vi "Test Copy from Pixmap Greyscale.vi"(8 "error in (no error)":errorcluster, 11 "Test Case In":refnum<class "Image.lvclass">) -> (0 "error out":errorcluster, 3 "Test Case Out":refnum<class "Image.lvclass">)   [LabVIEW 2020, in "g_ar_toolkit.test.lvlib" / "Image.lvclass"]
uses:
  Image.lvclass
  C:/Program Files (x86)/National Instruments/LabVIEW 2020/vi.lib/Astemes/LUnit/Test Case.lvclass
  <vilib>/picture/picture.llb/imagedata.ctl
  <vilib>/Astemes/LUnit/Test Case.lvclass/Test Case.ctl
  2c93f62b-78d7-4b59-b27c-14bd701a5d71.vi
  8166983f-db3b-480f-a786-a958408166cb.vi
  03fde0f0-e029-4dad-9f9a-a95d25ce423a.vi
  3bb2986f-6074-4300-8ef6-a7ee1c3ba308.vi
  02fb1d00-84d2-4392-bb0c-78c1f80e642d.vi
  g_ar_toolkit.image/CreateEmptyImageGreyscale.vi
  g_ar_toolkit.image/CopyPixmapToImageOuptutMaskGreyscale.vi
  g_ar_toolkit.image/CopyPixmapToImageIgnoreMaskGreyscale.vi
  7f5bb767-9dbf-47d9-8f44-5f4901e96d00.vi
  e6d5ae8e-bd70-4c65-a769-b7cfb03e80c7.vi
  d454bffa-6717-48ab-b8d5-b1f03345aa55.vi
  g_ar_toolkit.image/CreateEmptyImageGreyscale.vi/6598b9e0-8a08-46f5-91fd-ca1b87217137.vi
  g_ar_toolkit.image/CopyPixmapToImageOuptutMaskGreyscale.vi/80b1166a-8c06-443b-b271-eb6a715622f7.vi
  g_ar_toolkit.image/CopyPixmapToImageIgnoreMaskGreyscale.vi/80b1166a-8c06-443b-b271-eb6a715622f7.vi
  <vilib>/Astemes/LUnit/Append Pass Result.vi
  <vilib>/Astemes/LUnit/Append Fail Result.vi
  <vilib>/Astemes/LUnit/Describe Comparison.vi
  <vilib>/Astemes/LUnit/Compare Variants.vi
  g_ar_toolkit.image/FixPixmapColourArraySize.vi
  <vilib>/Astemes/LUnit/Variant to string.vi
  g_ar_toolkit.image/Default8bitColourMap.vi
  <vilib>/Utility/colorconv.llb/Color to RGB.vi
  <vilib>/Utility/error.llb/Error Cluster From Error Code.vi
  <vilib>/Utility/Data Type/Get Type Information.vi
  <vilib>/Utility/LVClass/Get LV Class Name.vi
  g_ar_toolkit.image/g_ar_toolkit.image.lvlib
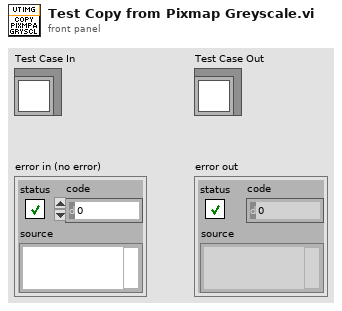
[diagram p1: front panel]
types:
  T1 = enum16{"8 Bit No Mask", "24 Bit No Mask", "32 Bit No Mask", "8 Bit Mask", "24 Bit Mask", "32 Bit Mask", "8 Pixels Wide Masked", "16 Pixels Wide Masked"}
  T2 = typedef "imagedata.ctl" = cluster{"image type":i32, "image depth":i32, "image":u8[], "mask":u8[], "colors":u32[], "Rectangle":cluster{"left":i16, "top":i16, "right":i16, "bottom":i16}}
  T3 = cluster{"8 No Mask":T2, "8 Mask":T2, "24 No Mask":T2, "24 Mask":T2, "32 No Mask":T2, "32 Mask":T2, "24 Mask - 8 wide":T2, "24 Mask - 16 wide":T2}
  T4 = cluster{"left":i16, "top":i16, "right":i16, "bottom":i16}
  T5 = enum16{"8 Bit No Mask", "24 Bit No Mask", "32 Bit No Mask", "8 Bit Mask", "24 Bit Mask", "32 Bit Mask", "8 Pixels Wide Masked", "16 Pixels Wide Masked"}[]
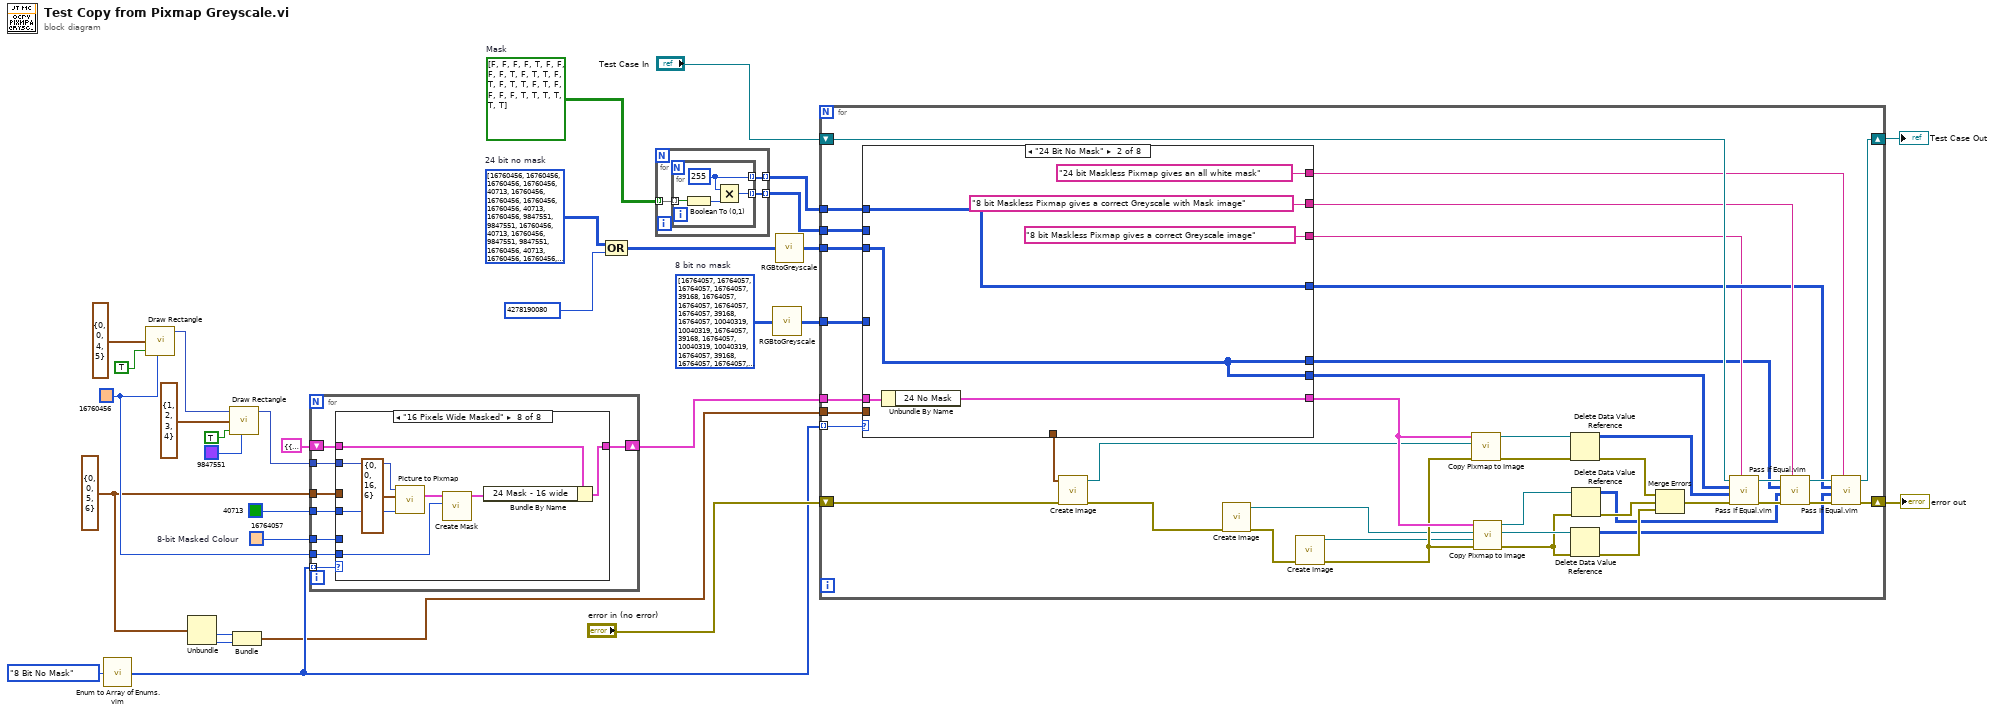
[diagram p0: block diagram]
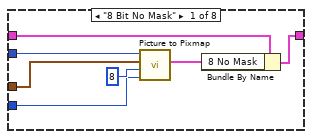
[diagram p2: hidden frame]
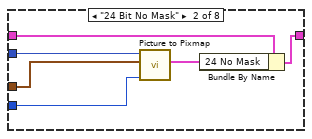
[diagram p3: hidden frame]
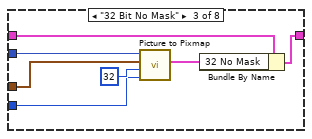
[diagram p4: hidden frame]
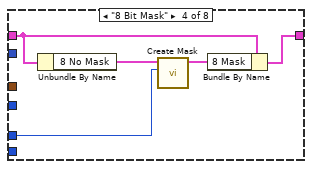
[diagram p5: hidden frame]
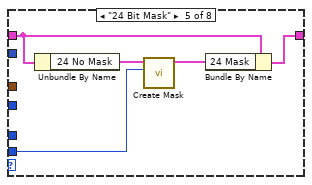
[diagram p6: hidden frame]
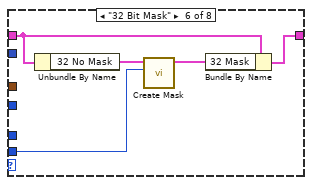
[diagram p7: hidden frame]
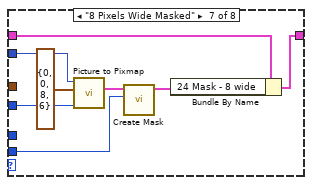
[diagram p8: hidden frame]
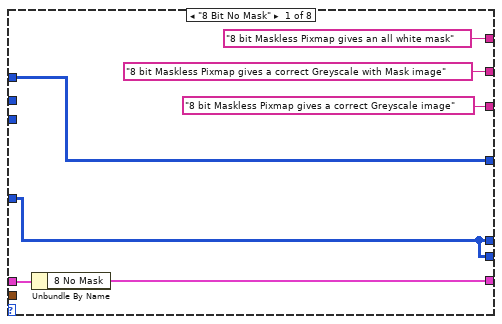
[diagram p9: hidden frame]
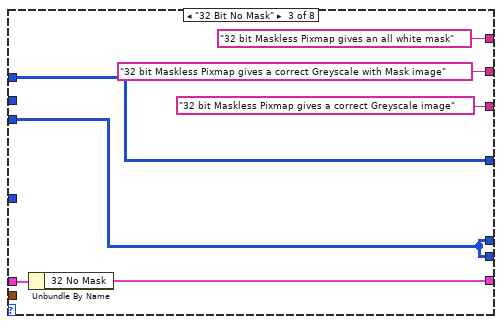
[diagram p10: hidden frame]
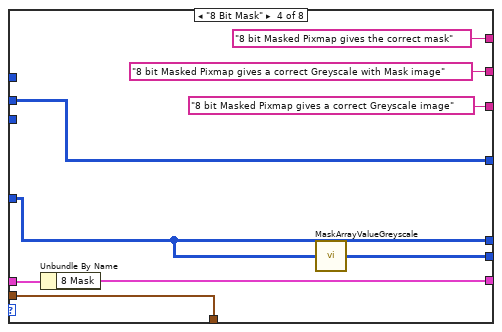
[diagram p11: hidden frame]
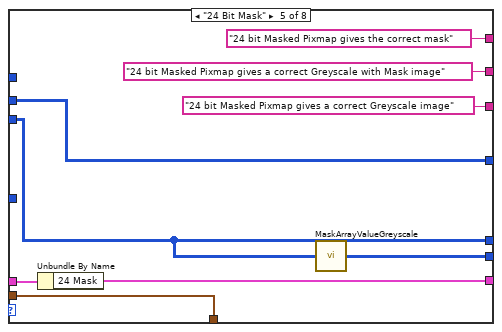
[diagram p12: hidden frame]
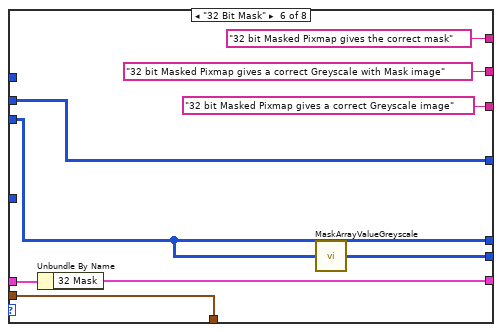
[diagram p13: hidden frame]
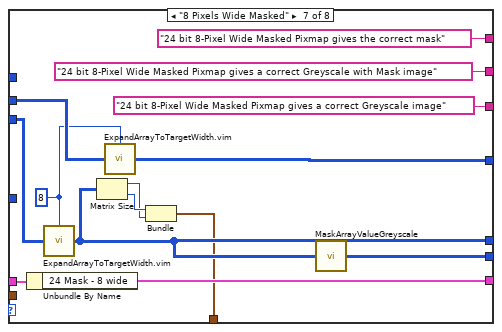
[diagram p14: hidden frame]
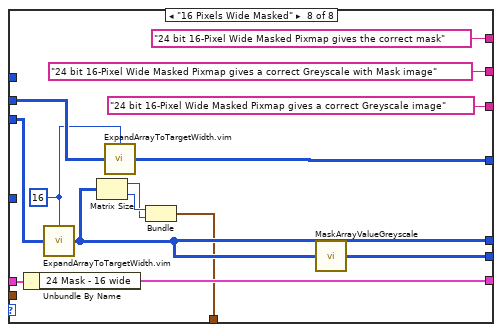
[diagram p15: hidden frame]
diagram:
  w5 = u32 16764057  # 8-bit Masked Colour
  w18 = bool[][] [[FALSE, FALSE, FALSE, FALSE, TRUE], [FALSE, FALSE, FALSE, FALSE, TRUE], [FALSE, TRUE, TRUE, FALSE, TRUE], [FALSE, TRUE, TRUE, FALSE, TRUE], [FALSE, FALSE, FALSE, FALSE, TRUE], [TRUE, TRUE, TRUE, TRUE, TRUE]]  # Mask
  w2 = u32[][] [[16764057, 16764057, 16764057, 16764057, 39168], [16764057, 16764057, 16764057, 16764057, 39168], [16764057, 10040319, 10040319, 16764057, 39168], [16764057, 10040319, 10040319, 16764057, 39168], [16764057, 16764057, 16764057, 16764057, 39168], [39168, 39168, 39168, 39168, 39168]]  # 8 bit no mask
  w21 = u32[][] [[16760456, 16760456, 16760456, 16760456, 40713], [16760456, 16760456, 16760456, 16760456, 40713], [16760456, 9847551, 9847551, 16760456, 40713], [16760456, 9847551, 9847551, 16760456, 40713], [16760456, 16760456, 16760456, 16760456, 40713], [40713, 40713, 40713, 40713, 40713]]  # 24 bit no mask
  w9 = T4 {"left"=0, "top"=0, "right"=5, "bottom"=6} ("rect")
  w12 = u32 16760456 ("color(black)")
  n1 = call "Enum to Array of Enums.vim"("enum"=T1."8 Bit No Mask") -> ("array of enums"=w16:T5)
  n2 = call <vilib>:"Draw Rectangle.vi"("rect"=T4 {"left"=0, "top"=0, "right"=4, "bottom"=5}, "fill?(F)"=TRUE, "color(black)"=w12) -> ("new picture"=w31:picture)  [unwired: 6 in]
  n3 = Unbundle(w9) -> ("right"=w8:i16, "bottom"=w7:i16)  [unwired: 2 out]
  n4 = call <vilib>:"Draw Rectangle.vi"("picture"=w31, "rect"=T4 {"left"=1, "top"=2, "right"=3, "bottom"=4}, "fill?(F)"=TRUE, "color(black)"=u32 9847551) -> ("new picture"=w13:picture)  [unwired: 5 in]
  n5 = Bundle("right"=w8, "bottom"=w7) -> (w6:cluster{"right":i16, "bottom":i16})  [unwired: 1 in]
  n6 = for {
    tunnel: w16 -> [w37] mode=indexing
    shift-right: [w38] -> w14
    shift-left: T3 {"8 No Mask"={"image type"=0, "image depth"=0, "image"=[], "mask"=[], "colors"=[], "Rectangle"={"left"=0, "top"=0, "right"=0, "bottom"=0}}, "8 Mask"={"image type"=0, "image depth"=0, "image"=[], "mask"=[], "colors"=[], "Rectangle"={"left"=0, "top"=0, "right"=0, "bottom"=0}}, "24 No Mask"={"image type"=0, "image depth"=0, "image"=[], "mask"=[], "colors"=[], "Rectangle"={"left"=0, "top"=0, "right"=0, "bottom"=0}}, "24 Mask"={"image type"=0, "image depth"=0, "image"=[], "mask"=[], "colors"=[], "Rectangle"={"left"=0, "top"=0, "right"=0, "bottom"=0}}, "32 No Mask"={"image type"=0, "image depth"=0, "image"=[], "mask"=[], "colors"=[], "Rectangle"={"left"=0, "top"=0, "right"=0, "bottom"=0}}, "32 Mask"={"image type"=0, "image depth"=0, "image"=[], "mask"=[], "colors"=[], "Rectangle"={"left"=0, "top"=0, "right"=0, "bottom"=0}}, "24 Mask - 8 wide"={"image type"=0, "image depth"=0, "image"=[], "mask"=[], "colors"=[], "Rectangle"={"left"=0, "top"=0, "right"=0, "bottom"=0}}, "24 Mask - 16 wide"={"image type"=0, "image depth"=0, "image"=[], "mask"=[], "colors"=[], "Rectangle"={"left"=0, "top"=0, "right"=0, "bottom"=0}}} ("output cluster") -> [w39]
    tunnel: w13 -> [w35]
    tunnel: w9 -> [w36]
    tunnel: u32 40713 ("Background Color") -> [w34]
    tunnel: w12 -> [w33]
    tunnel: w5 -> [w32]
    n7 = case shown="\"16 Pixels Wide Masked\"" w37 {
      tunnel: w39 -> [w46 w52 w59 w63 w68 w73 w82 w90]
      tunnel: [w45 w51 w58 w64 w69 w74 w81 w89] -> w38
      tunnel: w36 -> [w43 w50 w56 _ _ _ _ _]
      tunnel: w35 -> [w42 w49 w55 _ _ _ w78 w86]
      tunnel: w34 -> [w40 w47 w53 _ _ _ w77 w85]
      tunnel: w33 -> [_ _ _ _ w65 w70 w75 w83]
      tunnel: w32 -> [_ _ _ w60 _ _ _ _]
      frame "8 Bit No Mask" {
        n8 = call <vilib>:"Picture to Pixmap.vi"("Background Color"=w40, "depth"=8, "rect"=w43, "picture"=w42) -> ("image data"=w41:T2)  [unwired: 6 in, 1 out]
        n9 = Bundle By Name(cluster=w46, "8 No Mask"=w41) -> (w45:T3)
      }
      frame "24 Bit No Mask" {
        n10 = call <vilib>:"Picture to Pixmap.vi"("Background Color"=w47, "rect"=w50, "picture"=w49) -> ("image data"=w48:T2)  [unwired: 7 in, 1 out]
        n11 = Bundle By Name(cluster=w52, "24 No Mask"=w48) -> (w51:T3)
      }
      frame "32 Bit No Mask" {
        n12 = call <vilib>:"Picture to Pixmap.vi"("Background Color"=w53, "depth"=32, "rect"=w56, "picture"=w55) -> ("image data"=w54:T2)  [unwired: 6 in, 1 out]
        n13 = Bundle By Name(cluster=w59, "32 No Mask"=w54) -> (w58:T3)
      }
      frame "8 Bit Mask" {
        n14 = Unbundle By Name(w63) -> ("8 No Mask"=w62:T2)
        n15 = call <vilib>:"Create Mask.vi"("Mask Color (Black)"=w60, "image data"=w62) -> ("image data"=w61:T2)  [unwired: 9 in]
        n16 = Bundle By Name(cluster=w63, "8 Mask"=w61) -> (w64:T3)
      }
      frame "24 Bit Mask" {
        n17 = Unbundle By Name(w68) -> ("24 No Mask"=w67:T2)
        n18 = call <vilib>:"Create Mask.vi"("Mask Color (Black)"=w65, "image data"=w67) -> ("image data"=w66:T2)  [unwired: 9 in]
        n19 = Bundle By Name(cluster=w68, "24 Mask"=w66) -> (w69:T3)
      }
      frame "32 Bit Mask" {
        n20 = Unbundle By Name(w73) -> ("32 No Mask"=w72:T2)
        n21 = call <vilib>:"Create Mask.vi"("Mask Color (Black)"=w70, "image data"=w72) -> ("image data"=w71:T2)  [unwired: 9 in]
        n22 = Bundle By Name(cluster=w73, "32 Mask"=w71) -> (w74:T3)
      }
      frame "8 Pixels Wide Masked" {
        n23 = call <vilib>:"Picture to Pixmap.vi"("Background Color"=w77, "rect"=T4 {"left"=0, "top"=0, "right"=8, "bottom"=6}, "picture"=w78) -> ("image data"=w80:T2)  [unwired: 7 in, 1 out]
        n24 = call <vilib>:"Create Mask.vi"("Mask Color (Black)"=w75, "image data"=w80) -> ("image data"=w79:T2)  [unwired: 9 in]
        n25 = Bundle By Name(cluster=w82, "24 Mask - 8 wide"=w79) -> (w81:T3)
      }
      frame "16 Pixels Wide Masked" {
        n26 = call <vilib>:"Picture to Pixmap.vi"("Background Color"=w85, "rect"=T4 {"left"=0, "top"=0, "right"=16, "bottom"=6}, "picture"=w86) -> ("image data"=w88:T2)  [unwired: 7 in, 1 out]
        n27 = call <vilib>:"Create Mask.vi"("Mask Color (Black)"=w83, "image data"=w88) -> ("image data"=w87:T2)  [unwired: 9 in]
        n28 = Bundle By Name(cluster=w90, "24 Mask - 16 wide"=w87) -> (w89:T3)
      }
    }
  }
  n29 = Compound Arithmetic op=OR(w21, u32 4278190080) -> (w20:u32[][])
  n30 = for "Masks" {
    tunnel: w18 -> [w92] mode=indexing
    tunnel: [w93] -> w19 mode=indexing
    tunnel: [w91] -> w17 mode=indexing
    n31 = for {
      tunnel: [w96] -> w93 mode=indexing
      tunnel: w92 -> [w97] mode=indexing
      tunnel: [w95] -> w91 mode=indexing
      w96 = u8 255 ("unsigned 8bit integer")
      n32 = Boolean To (0,1)(Boolean=w97) -> (0, 1=w94:i16)
      n33 = Multiply(x=w96, y=w94) -> (x*y=w95:u8)
    }
  }
  n34 = call "RGBtoGreyscale.vi"("RBG"=w2) -> ("Greyscale"=w3:u8[][])
  n35 = call "RGBtoGreyscale.vi"("RBG"=w20) -> ("Greyscale"=w1:u8[][])
  n36 = for {
    tunnel: w14 -> [w138]
    tunnel: w16 -> [w132] mode=indexing
    shift-right: [w123] -> w22
    shift-left: "error in (no error)" -> [w115]
    shift-right: [w122] -> w25
    shift-left: "Test Case In" -> [w131]
    tunnel: w1 -> [w116]
    tunnel: w3 -> [w119]
    tunnel: w19 -> [w112]
    tunnel: w17 -> [w111]
    tunnel: w6 -> [w106]
    n37 = case shown="\"24 Bit No Mask\"" w132 {
      tunnel: w138 -> [w145 w152 w159 w168 w177 w186 w200 w214]
      tunnel: [w144 w151 w158 w167 w176 w185 w199 w213] -> w137
      tunnel: ["8 bit Maskless Pixmap gives an all white mask" ("Description") "24 bit Maskless Pixmap gives an all white mask" ("Description") "32 bit Maskless Pixmap gives an all white mask" ("Description") "8 bit Masked Pixmap gives the correct mask" ("Description") "24 bit Masked Pixmap gives the correct mask" ("Description") "32 bit Masked Pixmap gives the correct mask" ("Description") "24 bit 8-Pixel Wide Masked Pixmap gives the correct mask" ("Description") "24 bit 16-Pixel Wide Masked Pixmap gives the correct mask" ("Description")] -> w121
      tunnel: ["8 bit Maskless Pixmap gives a correct Greyscale with Mask image" ("Description") "8 bit Maskless Pixmap gives a correct Greyscale with Mask image" ("Description") "32 bit Maskless Pixmap gives a correct Greyscale with Mask image" ("Description") "8 bit Masked Pixmap gives a correct Greyscale with Mask image" ("Description") "24 bit Masked Pixmap gives a correct Greyscale with Mask image" ("Description") "32 bit Masked Pixmap gives a correct Greyscale with Mask image" ("Description") "24 bit 8-Pixel Wide Masked Pixmap gives a correct Greyscale with Mask image" ("Description") "24 bit 16-Pixel Wide Masked Pixmap gives a correct Greyscale with Mask image" ("Description")] -> w120
      tunnel: [w141 w146 w153 w161 w171 w180 w195 w209] -> w99
      tunnel: w119 -> [w141 _ _ w164 _ _ _ _]
      tunnel: [w141 w146 w153 w164 w169 w178 w190 w204] -> w100
      tunnel: [w139 w147 w154 w160 w170 w179 w192 w206] -> w118
      tunnel: ["8 bit Maskless Pixmap gives a correct Greyscale image" ("Description") "8 bit Maskless Pixmap gives a correct Greyscale image" ("Description") "32 bit Maskless Pixmap gives a correct Greyscale image" ("Description") "8 bit Masked Pixmap gives a correct Greyscale image" ("Description") "24 bit Masked Pixmap gives a correct Greyscale image" ("Description") "32 bit Masked Pixmap gives a correct Greyscale image" ("Description") "24 bit 8-Pixel Wide Masked Pixmap gives a correct Greyscale image" ("Description") "24 bit 16-Pixel Wide Masked Pixmap gives a correct Greyscale image" ("Description")] -> w117
      tunnel: w116 -> [_ w146 w153 _ w169 w178 w193 w207]
      tunnel: w112 -> [w139 w147 w154 _ _ _ _ _]
      tunnel: w111 -> [_ _ _ w160 w170 w179 w194 w208]
      tunnel: [_ _ _ w162 w172 w181 w187 w201] -> w107
      tunnel: w106 -> [_ _ _ w162 w172 w181 _ _]
      frame "8 Bit No Mask" {
        n38 = Unbundle By Name(w145) -> ("8 No Mask"=w144:T2)
      }
      frame "24 Bit No Mask" {
        n39 = Unbundle By Name(w152) -> ("24 No Mask"=w151:T2)
      }
      frame "32 Bit No Mask" {
        n40 = Unbundle By Name(w159) -> ("32 No Mask"=w158:T2)
      }
      frame "8 Bit Mask" {
        n41 = Unbundle By Name(w168) -> ("8 Mask"=w167:T2)
        n42 = call "MaskArrayValueGreyscale.vi"("Array In"=w164) -> ("Array out"=w161:u8[][])
      }
      frame "24 Bit Mask" {
        n43 = Unbundle By Name(w177) -> ("24 Mask"=w176:T2)
        n44 = call "MaskArrayValueGreyscale.vi"("Array In"=w169) -> ("Array out"=w171:u8[][])
      }
      frame "32 Bit Mask" {
        n45 = Unbundle By Name(w186) -> ("32 Mask"=w185:T2)
        n46 = call "MaskArrayValueGreyscale.vi"("Array In"=w178) -> ("Array out"=w180:u8[][])
      }
      frame "8 Pixels Wide Masked" {
        w191 = 8 ("Target Width")
        n47 = Unbundle By Name(w200) -> ("24 Mask - 8 wide"=w199:T2)
        n48 = call "ExpandArrayToTargetWidth.vim"("Array in"=w193, "Target Width"=w191) -> ("Array out"=w190:u8[][])
        n49 = Matrix Size(0:w190) -> (1:w188:i32, 2:w189:i32)
        n50 = call "ExpandArrayToTargetWidth.vim"("Array in"=w194, "Target Width"=w191) -> ("Array out"=w192:u8[][])
        n51 = Bundle("matrix"=w189, "number of columns"=w188) -> (w187:cluster{"matrix":i32, "number of columns":i32})  [unwired: 1 in]
        n52 = call "MaskArrayValueGreyscale.vi"("Array In"=w190) -> ("Array out"=w195:u8[][])
      }
      frame "16 Pixels Wide Masked" {
        w205 = 16 ("Target Width")
        n53 = Unbundle By Name(w214) -> ("24 Mask - 16 wide"=w213:T2)
        n54 = call "ExpandArrayToTargetWidth.vim"("Array in"=w207, "Target Width"=w205) -> ("Array out"=w204:u8[][])
        n55 = Matrix Size(0:w204) -> (1:w202:i32, 2:w203:i32)
        n56 = call "ExpandArrayToTargetWidth.vim"("Array in"=w208, "Target Width"=w205) -> ("Array out"=w206:u8[][])
        n57 = Bundle("matrix"=w203, "number of columns"=w202) -> (w201:cluster{"matrix":i32, "number of columns":i32})  [unwired: 1 in]
        n58 = call "MaskArrayValueGreyscale.vi"("Array In"=w204) -> ("Array out"=w209:u8[][])
      }
    }
    n59 = call-poly "Create Image.vi"("error in (no error)"=w115, "Preallocated Image Size (Default 0,0)"=w107) -> ("error out"=w114:errorcluster, "New Greyscale Image"=w113:refnum<data-value>)  [unwired: 8 in]
    n60 = call-poly "Create Image.vi"("error in (no error)"=w114) -> ("error out"=w110:errorcluster, "New Greyscale Image"=w108:refnum<data-value>)  [unwired: 9 in]
    n61 = call-poly "Create Image.vi"("error in (no error)"=w110) -> ("error out"=w136:errorcluster, "New Greyscale Image"=w109:refnum<data-value>)  [unwired: 9 in]
    n62 = call-poly "Copy Pixmap to Image.vi"("error in (no error)"=w136, "Greyscale Image Destination"=w113, "Pixmap Image Data"=w137) -> ("error out"=w102:errorcluster, "Greyscale Image Destination (duplicate)"=w101:refnum<data-value>)  [unwired: 7 in]
    n63 = call-poly "Copy Pixmap to Image.vi"("error in (no error)"=w136, "Greyscale Image Mask"=w109, "Greyscale Image Destination"=w108, "Pixmap Image Data"=w137) -> ("error out"=w104:errorcluster, "Greyscale Image Mask (duplicate)"=w105:refnum<data-value>, "Greyscale Image Destination (duplicate)"=w103:refnum<data-value>)  [unwired: 5 in]
    n64 = Delete Data Value Reference(data value reference=w101, error in=w102) -> (data value=w98:u8[][], error out=w135:errorcluster)
    n65 = Delete Data Value Reference(data value reference=w105, error in=w104) -> (data value=w125:u8[][], error out=w133:errorcluster)
    n66 = Delete Data Value Reference(data value reference=w103, error in=w104) -> (data value=w126:u8[][], error out=w134:errorcluster)
    n67 = Merge Errors(w135, w134, w133) -> (w124:errorcluster)
    n68 = call "Pass If Equal.vim"("Description"=w117, "error in (no error)"=w124, "Actual"=w98, "Expected"=w99, "LUnit Test Case In"=w131) -> ("error out"=w128:errorcluster, "LUnit Test Case Out"=w130:refnum<class "Image.lvclass">)  [unwired: 5 in]
    n69 = call "Pass If Equal.vim"("Description"=w120, "error in (no error)"=w128, "Actual"=w126, "Expected"=w100, "LUnit Test Case In"=w130) -> ("error out"=w127:errorcluster, "LUnit Test Case Out"=w129:refnum<class "Image.lvclass">)  [unwired: 5 in]
    n70 = call "Pass If Equal.vim"("Description"=w121, "error in (no error)"=w127, "Actual"=w125, "Expected"=w118, "LUnit Test Case In"=w129) -> ("error out"=w123:errorcluster, "LUnit Test Case Out"=w122:refnum<class "Image.lvclass">)  [unwired: 5 in]
  }
  "error out" <- w22
  "Test Case Out" <- w25
